vi "Create Mixed IO.vi"(8 "error in":errorcluster, 11 "6509 in":refnum<class "6509.lvclass">) -> (0 "error out":errorcluster, 3 "6509 out":refnum<class "6509.lvclass">)   [LabVIEW 2019, in "6509.lvlib" / "6509.lvclass"]
uses:
  Library/6509.lvclass
  C:/Users/Public/Documents/Development/builds/Instruments/DIG_IO.lvlibp/Library/DIG_IO.lvclass
  Library/6509.lvclass/6509.ctl
  builds/Instruments/DIG_IO.lvlibp/Accessors/Read BankDefs.vi
  <resource>/objmgr/daqmx.rc
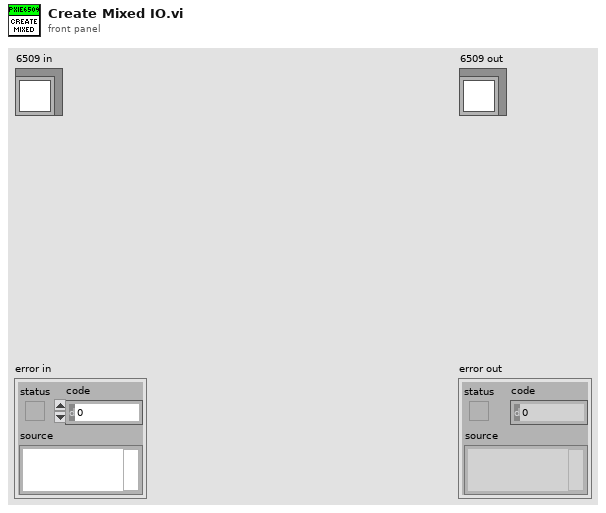
[diagram p1: front panel]
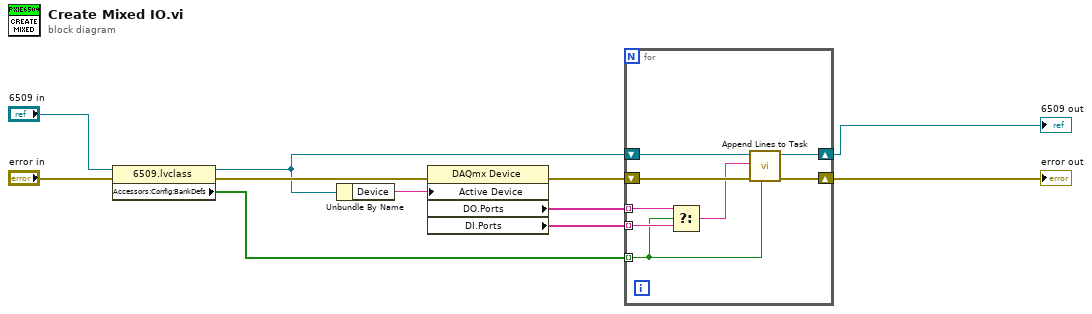
[diagram p0: block diagram]
diagram:
  n1 = property class="6509.lvclass"(reference="6509 in", error in="error in") -> (reference out=w2:refnum<class "6509.lvclass">, error out=w4:errorcluster, "Accessors:Config:BankDefs"=w1:bool[])
  n2 = Unbundle By Name(w2) -> ("Device"=w10:tag)
  n3 = property class="DAQmx Device"(error in=w4, "Active Device"=w10) -> (error out=w9:errorcluster, "DO.Ports"=w6:tag[], "DI.Ports"=w5:tag[])  [unwired: 1 in, 1 out]
  n4 = for {
    shift-right: [w18] -> w8
    shift-left: w9 -> [w19]
    shift-right: [w16] -> w7
    shift-left: w2 -> [w17]
    tunnel: w6 -> [w15] mode=indexing
    tunnel: w5 -> [w14] mode=indexing
    tunnel: w1 -> [w12] mode=indexing
    n5 = Select(t=w15, s=w12, f=w14) -> (s? t:f=w13:tag)
    n6 = call "Append Lines to Task.vi"("Control"=w12, "error in"=w19, "lines"=w13, "6509 in"=w17) -> ("error out"=w18:errorcluster, "6509 out"=w16:refnum<class "6509.lvclass">)  [unwired: 6 in]
  }
  "error out" <- w8
  "6509 out" <- w7
